vi "Archive Message Loop.vi"(8 "error in (no error)":errorcluster, 11 "Message Queues":T1) -> (0 "error out":errorcluster)   [LabVIEW 2024]
doc: "This is a working thread of the server and is responsible for data archiving."
uses:
  Shared/Message Queue/Server Message Queues.ctl
  Shared/Message Queue/Message Cluster.ctl
  Controls/Server/System Configuration.ctl
  Controls/Server/Subsystem Configuration.ctl
  Timer/Timer Parameter.ctl
  Shared/Message Queue.lvlib
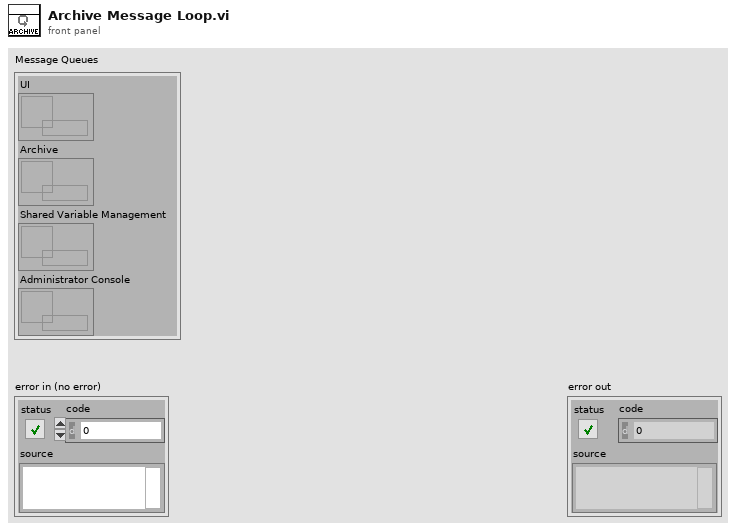
[diagram p1: front panel]
types:
  T1 = typedef "Message Queue.lvlib/Server Message Queues.ctl" = cluster{"UI":refnum<queue>, "Archive":refnum<queue>, "Shared Variable Management":refnum<queue>, "Administrator Console":refnum<queue>}
  T2 = typedef "System Configuration.ctl" = cluster{"Name":string, "Description":string, "Logging Computer Name":string, "Logging Database Name":string, "Logging Database Path":path, "Archive Computer Name":string, "Archive Database Name":string, "Archive Database Path":path, "Lifespan (days)":u32, "Archive Enabled":bool, "Archive Interval (hours)":u32, "Subsystems":T3[]}
  T3 = typedef "Subsystem Configuration.ctl" = cluster{"Name":string, "Root URL":refnum<k21>}
  T4 = typedef "Timer Parameter.ctl" = cluster{"Index":u32, "Value":variant}
  T5 = typedef "Timer Handler.ctl" = cluster{"Start Event":refnum<user-event>, "Stop Event":refnum<user-event>, "Exit Event":refnum<user-event>, "Timer Index":u32}
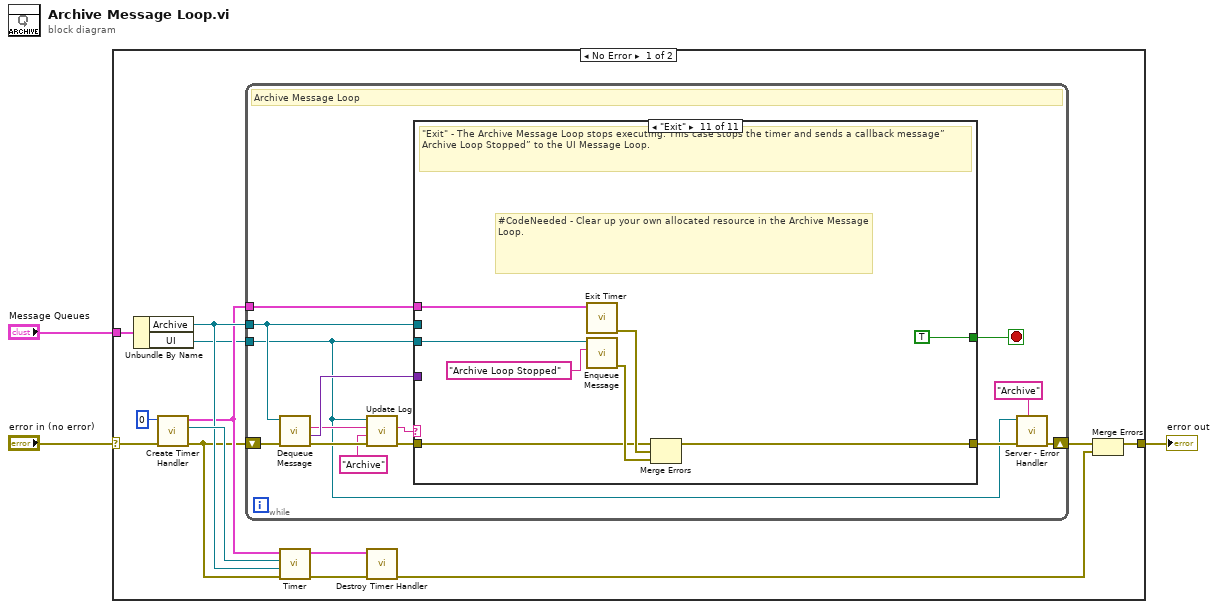
[diagram p0: block diagram]
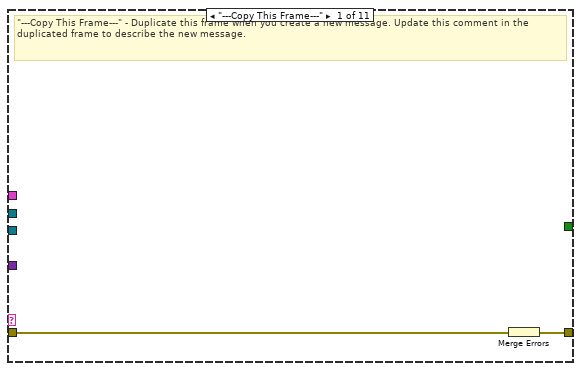
[diagram p2: hidden frame]
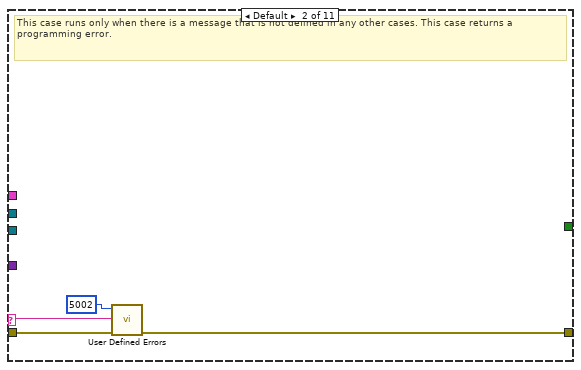
[diagram p3: hidden frame]
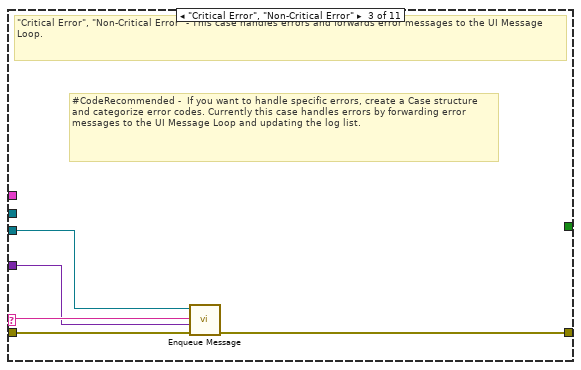
[diagram p4: hidden frame]
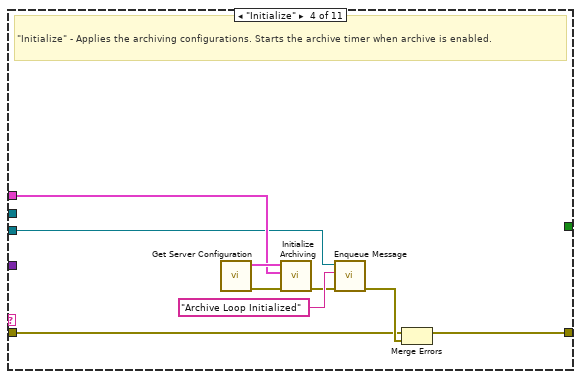
[diagram p5: hidden frame]
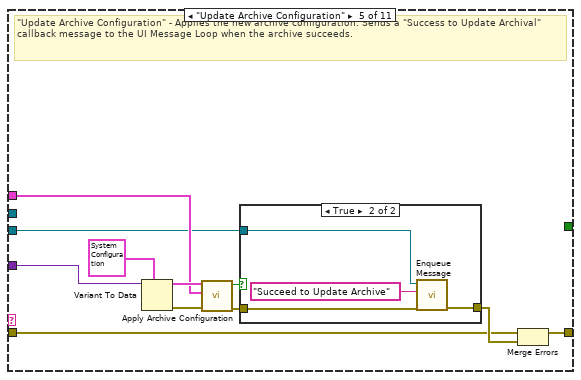
[diagram p6: hidden frame]
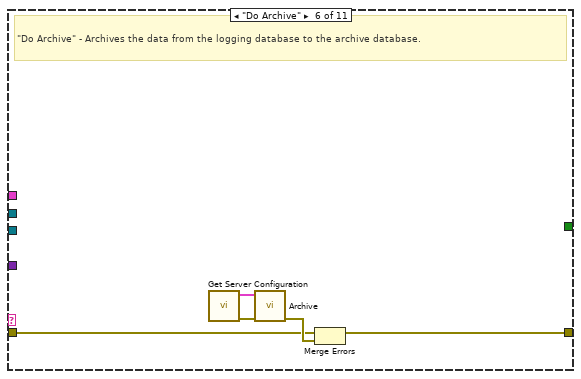
[diagram p8: hidden frame]
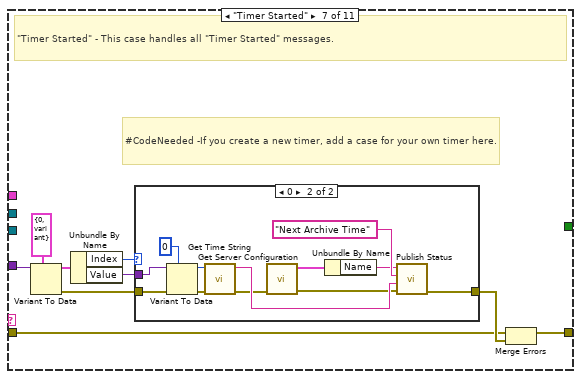
[diagram p9: hidden frame]
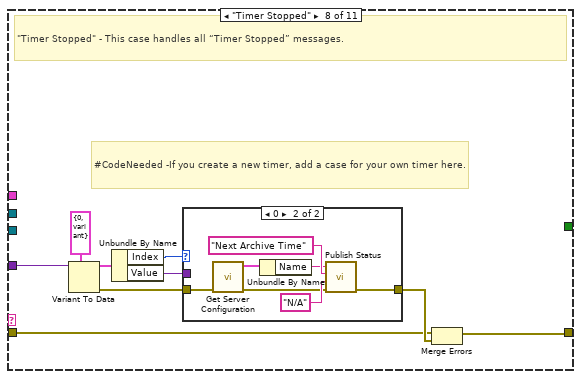
[diagram p11: hidden frame]
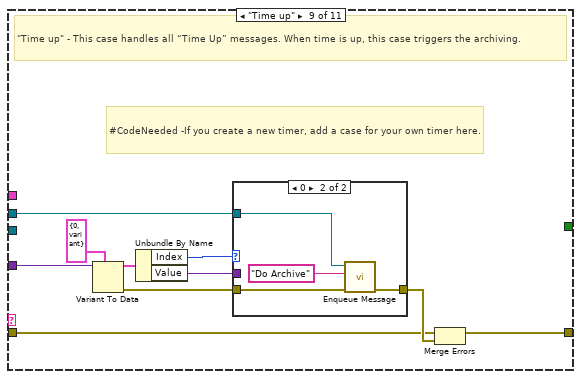
[diagram p13: hidden frame]
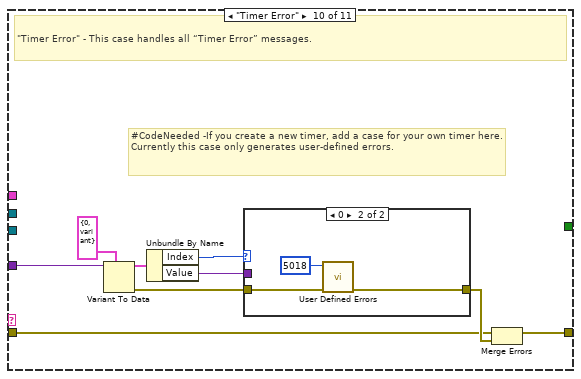
[diagram p15: hidden frame]
diagram:
  n1 = case shown="No Error" "error in (no error)" {
    selector: "error in (no error)" -> [w16 w147]
    tunnel: [w13 w147] -> w2
    tunnel: "Message Queues" -> [w4 _]
    frame No Error {
      n2 = Unbundle By Name(w4) -> ("Archive"=w10:refnum<queue>, "UI"=w5:refnum<queue>)
      n3 = call "Create Timer Handler.vi"("error in (no error)"=w16, "Timer Index"=u32 0) -> ("error out"=w6:errorcluster, "Event Registration Refnum"=w11:refnum<event-registration>, "Timer Handler"=w8:T5)  [unwired: 7 in]
      n4 = while {
        tunnel: w10 -> [w18]
        shift-right: [w25] -> w14
        shift-left: w6 -> [w29]
        tunnel: w5 -> [w17]
        tunnel: w8 -> [w19]
        stop <- w30 stop-if-true
        # "Archive Message Loop"
        n5 = call "Dequeue Message.vi"("error in (no error)"=w29, "Message Queue"=w18) -> ("error out"=w27:errorcluster, "Message Data"=w28:variant, "Message"=w23:string)  [unwired: 6 in, 1 out]
        n6 = call "Update Log.vi"("error in (no error)"=w27, "Component"="Archive", "Status"=w23, "UI Message Queue"=w17) -> ("error out"=w26:errorcluster, "dup Status"=w22:string)  [unwired: 5 in, 1 out]
        n7 = case "Message Cases" shown="\"Exit\"" w22 {
          selector: w22 -> [_ w34 w41 _ _ _ _ _ _ _ _]
          tunnel: [w32 w36 w38 w48 w55 w68 w75 w96 w114 w128 w145] -> w24
          tunnel: [_ _ _ _ _ _ _ _ _ _ TRUE] -> w30
          tunnel: w28 -> [_ _ w40 _ w57 _ w74 w97 w118 w129 _]
          tunnel: w26 -> [w31 w33 w39 w42 w51 w67 w72 w94 w111 w126 w139]
          tunnel: w19 -> [_ _ _ w44 w56 _ _ _ _ _ w143]
          tunnel: w18 -> [_ _ _ _ _ _ _ _ w113 _ _]
          tunnel: w17 -> [_ _ w37 w43 w53 _ _ _ _ _ w142]
          frame "---Copy This Frame---" {
            # "\"---Copy This Frame---\" - Duplicate this frame when you create a new message. Update this comment in the duplicated frame to describe the new message."
            n8 = Merge Errors(w31) -> (w32:errorcluster)
          }
          frame Default {
            # "This case runs only when there is a message that is not defined in any other cases. This case returns a programming error."
            n9 = call "User Defined Errors.vi"("error in (no error)"=w33, "Parameter 1"=w34, "Error Code (0)"=5002 ("error code (0)")) -> ("error out"=w36:errorcluster)  [unwired: 8 in]
          }
          frame "Critical Error", "Non-Critical Error" {
            # "#CodeRecommended -  If you want to handle specific errors, create a Case structure and categorize error codes. Currently this case handles errors by forwarding error messages to the UI Message Loop and updating the log list."
            # "\"Critical Error\", \"Non-Critical Error\" - This case handles errors and forwards error messages to the UI Message Loop."
            n10 = call "Enqueue Message.vi"("error in (no error)"=w39, "Message Data"=w40, "Message"=w41, "Message Queue"=w37) -> ("error out"=w38:errorcluster)  [unwired: 6 in, 1 out]
          }
          frame "Initialize" {
            # "\"Initialize\" - Applies the archiving configurations. Starts the archive timer when archive is enabled."
            n11 = call "Get Server Configuration.vi"() -> ("error out"=w46:errorcluster, "System Configuration"=w45:T2)  [unwired: 9 in, 1 out]
            n12 = call "Initialize Archiving.vi"("error in (no error)"=w46, "Timer Handler"=w44, "System Configuration"=w45) -> ("error out"=w49:errorcluster)  [unwired: 7 in, 1 out]
            n13 = call "Enqueue Message.vi"("error in (no error)"=w49, "Message"="Archive Loop Initialized", "Message Queue"=w43) -> ("error out"=w47:errorcluster)  [unwired: 7 in, 1 out]
            n14 = Merge Errors(w42, w47) -> (w48:errorcluster)
          }
          frame "Update Archive Configuration" {
            # "\"Update Archive Configuration\" - Applies the new archive configuration. Sends a \"Success to Update Archival\" callback message to the UI Message Loop when the archive succeeds."
            n15 = Variant To Data(type=T2 {"Name"="", "Description"="", "Logging Computer Name"="", "Logging Database Name"="", "Logging Database Path"=path "", "Archive Computer Name"="", "Archive Database Name"="", "Archive Database Path"=path "", "Lifespan (days)"=0, "Archive Enabled"=FALSE, "Archive Interval (hours)"=0, "Subsystems"=[]} ("System Configuration"), Variant=w57) -> (data=w60:T2, error out=w61:errorcluster)  [unwired: 1 in]
            n16 = call "Apply Archive Configuration.vi"("error in (no error)"=w61, "Timer Handler"=w56, "System Configuration"=w60) -> ("error out"=w58:errorcluster, "Succeed?"=w52:bool)  [unwired: 7 in]
            n17 = case shown="True" w52 {
              tunnel: w58 -> [w62 w65]
              tunnel: [w62 w64] -> w54
              tunnel: w53 -> [_ w63]
              frame False {
              }
              frame True {
                n18 = call "Enqueue Message.vi"("error in (no error)"=w65, "Message"="Succeed to Update Archive", "Message Queue"=w63) -> ("error out"=w64:errorcluster)  [unwired: 7 in, 1 out]
              }
            }
            n19 = Merge Errors(w51, w54) -> (w55:errorcluster)
          }
          frame "Do Archive" {
            # "\"Do Archive\" - Archives the data from the logging database to the archive database."
            n20 = call "Get Server Configuration.vi"() -> ("error out"=w70:errorcluster, "System Configuration"=w71:T2)  [unwired: 9 in, 1 out]
            n21 = call "Archive.vi"("error in (no error)"=w70, "System Configuration"=w71) -> ("error out"=w69:errorcluster)  [unwired: 9 in]
            n22 = Merge Errors(w67, w69) -> (w68:errorcluster)
          }
          frame "Timer Started" {
            # "#CodeNeeded -If you create a new timer, add a case for your own timer here."
            # "\"Timer Started\" - This case handles all \"Timer Started\" messages."
            n23 = Variant To Data(type=T4 {"Index"=0, "Value"=variant} ("Alarm Parameter"), Variant=w74) -> (data=w79:T4, error out=w77:errorcluster)  [unwired: 1 in]
            n24 = Unbundle By Name(w79) -> ("Index"=w78:u32, "Value"=w76:variant)
            n25 = case shown="0" w78 {
              tunnel: w77 -> [w81 w86]
              tunnel: w76 -> [_ w87]
              tunnel: [w81 w92] -> w73
              frame Default {
              }
              frame 0 {
                n26 = Variant To Data(error in=w86, type=u32 0 ("Index"), Variant=w87) -> (data=w84:u32, error out=w85:errorcluster)
                n27 = call "Get Time String.vi"("error in (no error)"=w85, "Offset (s)"=w84) -> ("error out"=w83:errorcluster, "Time String"=w91:string)  [unwired: 8 in]
                n28 = call "Get Server Configuration.vi"("error in (no error)"=w83) -> ("error out"=w82:errorcluster, "System Configuration"=w89:T2)  [unwired: 8 in, 1 out]
                n29 = Unbundle By Name(w89) -> ("Name"=w88:string)
                n30 = call "Publish Status.vi"("error in (no error)"=w82, "Value"=w91, "Parameter"="Next Archive Time", "System Name"=w88) -> ("error out"=w92:errorcluster)  [unwired: 7 in]
              }
            }
            n31 = Merge Errors(w72, w73) -> (w75:errorcluster)
          }
          frame "Timer Stopped" {
            # "#CodeNeeded -If you create a new timer, add a case for your own timer here."
            # "\"Timer Stopped\" - This case handles all “Timer Stopped” messages."
            n32 = Variant To Data(type=T4 {"Index"=0, "Value"=variant} ("Alarm Parameter"), Variant=w97) -> (data=w101:T4, error out=w99:errorcluster)  [unwired: 1 in]
            n33 = Unbundle By Name(w101) -> ("Index"=w100:u32, "Value"=w98:variant)
            n34 = case shown="0" w100 {
              tunnel: w99 -> [w103 w106]
              tunnel: w98 -> [_ _]
              tunnel: [w103 w108] -> w95
              frame Default {
              }
              frame 0 {
                n35 = call "Get Server Configuration.vi"("error in (no error)"=w106) -> ("error out"=w104:errorcluster, "System Configuration"=w107:T2)  [unwired: 8 in, 1 out]
                n36 = Unbundle By Name(w107) -> ("Name"=w105:string)
                n37 = call "Publish Status.vi"("error in (no error)"=w104, "Value"="N/A" ("Message"), "Parameter"="Next Archive Time", "System Name"=w105) -> ("error out"=w108:errorcluster)  [unwired: 7 in]
              }
            }
            n38 = Merge Errors(w94, w95) -> (w96:errorcluster)
          }
          frame "Time up" {
            # "#CodeNeeded -If you create a new timer, add a case for your own timer here."
            # "\"Time up\" - This case handles all “Time Up” messages. When time is up, this case triggers the archiving."
            n39 = Variant To Data(type=T4 {"Index"=0, "Value"=variant} ("Alarm Parameter"), Variant=w118) -> (data=w119:T4, error out=w115:errorcluster)  [unwired: 1 in]
            n40 = Unbundle By Name(w119) -> ("Index"=w117:u32, "Value"=w116:variant)
            n41 = case shown="0" w117 {
              tunnel: w116 -> [_ _]
              tunnel: w115 -> [w121 w124]
              tunnel: w113 -> [_ w123]
              tunnel: [w121 w122] -> w112
              frame Default {
              }
              frame 0 {
                n42 = call "Enqueue Message.vi"("error in (no error)"=w124, "Message"="Do Archive", "Message Queue"=w123) -> ("error out"=w122:errorcluster)  [unwired: 7 in, 1 out]
              }
            }
            n43 = Merge Errors(w111, w112) -> (w114:errorcluster)
          }
          frame "Timer Error" {
            # "#CodeNeeded -If you create a new timer, add a case for your own timer here. Currently this case only generates user-defined errors."
            # "\"Timer Error\" - This case handles all “Timer Error” messages."
            n44 = Variant To Data(type=T4 {"Index"=0, "Value"=variant} ("Alarm Parameter"), Variant=w129) -> (data=w133:T4, error out=w130:errorcluster)  [unwired: 1 in]
            n45 = Unbundle By Name(w133) -> ("Index"=w132:u32, "Value"=w131:variant)
            n46 = case shown="0" w132 {
              tunnel: w131 -> [_ _]
              tunnel: w130 -> [w135 w137]
              tunnel: [w135 w136] -> w127
              frame Default {
              }
              frame 0 {
                n47 = call "User Defined Errors.vi"("error in (no error)"=w137, "Error Code (0)"=5018 ("error code (0)")) -> ("error out"=w136:errorcluster)  [unwired: 9 in]
              }
            }
            n48 = Merge Errors(w126, w127) -> (w128:errorcluster)
          }
          frame "Exit" {
            # "#CodeNeeded - Clear up your own allocated resource in the Archive Message Loop."
            # "\"Exit\" - The Archive Message Loop stops executing. This case stops the timer and sends a callback message” Archive Loop Stopped” to the UI Message Loop."
            n49 = call "Exit Timer.vi"("Timer Handler"=w143) -> ("error out"=w141:errorcluster)  [unwired: 10 in]
            n50 = call "Enqueue Message.vi"("Message"="Archive Loop Stopped", "Message Queue"=w142) -> ("error out"=w140:errorcluster)  [unwired: 8 in, 1 out]
            n51 = Merge Errors(w139, w141, w140) -> (w145:errorcluster)
          }
        }
        n52 = call "Server - Error Handler.vi"("Component"="Archive", "error in (no error)"=w24, "Message Queue"=w17) -> ("error out"=w25:errorcluster)  [unwired: 8 in]
      }
      n53 = call "Timer.vi"("error in (no error)"=w6, "Message Queue"=w10, "Event Registration Refnum"=w11, "Timer Handler"=w8) -> ("error out"=w9:errorcluster, "dup Timer Handler"=w7:T5)  [unwired: 6 in]
      n54 = call "Destroy Timer Handler.vi"("error in (no error)"=w9, "Timer Handler"=w7) -> ("error out"=w12:errorcluster)  [unwired: 9 in]
      n55 = Merge Errors(w14, w12) -> (w13:errorcluster)
    }
    frame Error {
    }
  }
  "error out" <- w2
